vi "ccd_livescan.vi"(8 "Or, read path automatically from:":path, 9 "Manual save directory":string, 10 "Manual save path":path, 11 "Manual (up) or automatic (down)":bool) -> ()   [LabVIEW 2009]
uses:
  <vilib>/vision/NI_Vision_Development_Module.lvlib
panel:
  in  "STOP":bool
  out "Log":string
  out "RFPI":dbl
  out "YFPI":dbl
  out "GFPI":dbl
  out "CI":dbl
  out "RI":dbl
  out "GI":dbl
  out "BF":dbl
  out "Loop counter (not important)":i32
  out "Live saturation image":T1(plugin-control)
  out "Live image":T1(plugin-control)
  out "Histogram graph":T2(graph)
  out "Snapshots":string
  in  "Custom snapshot":bool
  in  "BF snapshot":bool
  in  "RFP snapshot":bool
  in  "YFP snapshot":bool
  in  "GFP snapshot":bool
  in  "Red snapshot":bool
  in  "Green snapshot":bool
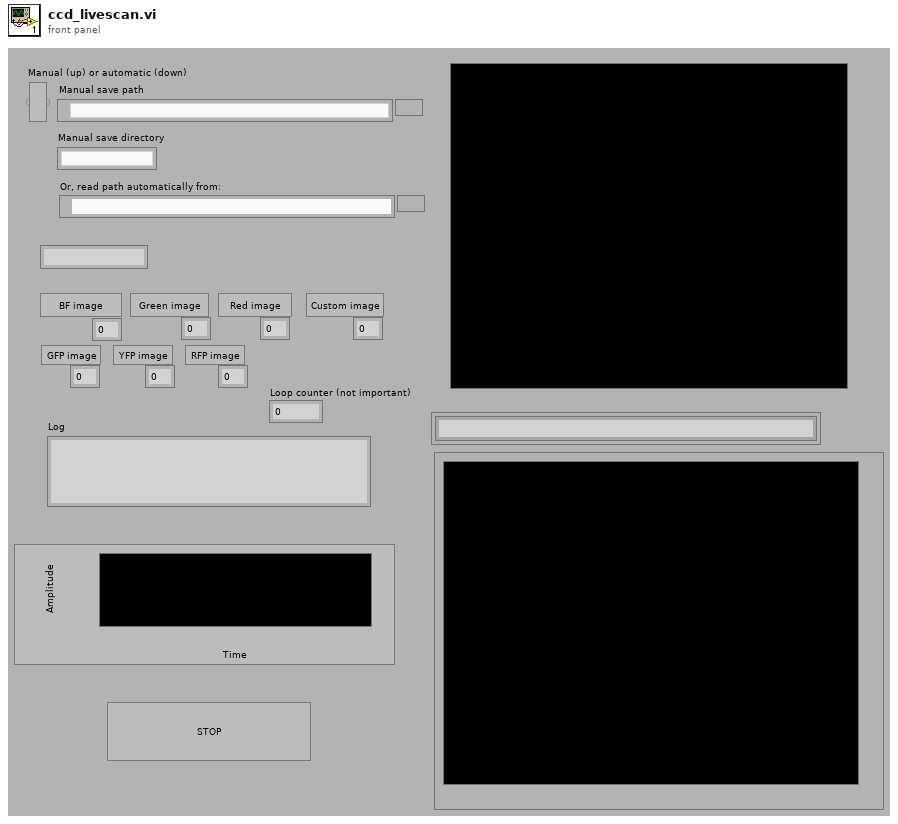
[diagram p1: front panel]
types:
  T1 = typedef "IMAQ Image.ctl" = refnum<image>
  T2 = cluster{"Starting Value":sgl, "Incremental Value":sgl, "Histogram":u32[]}
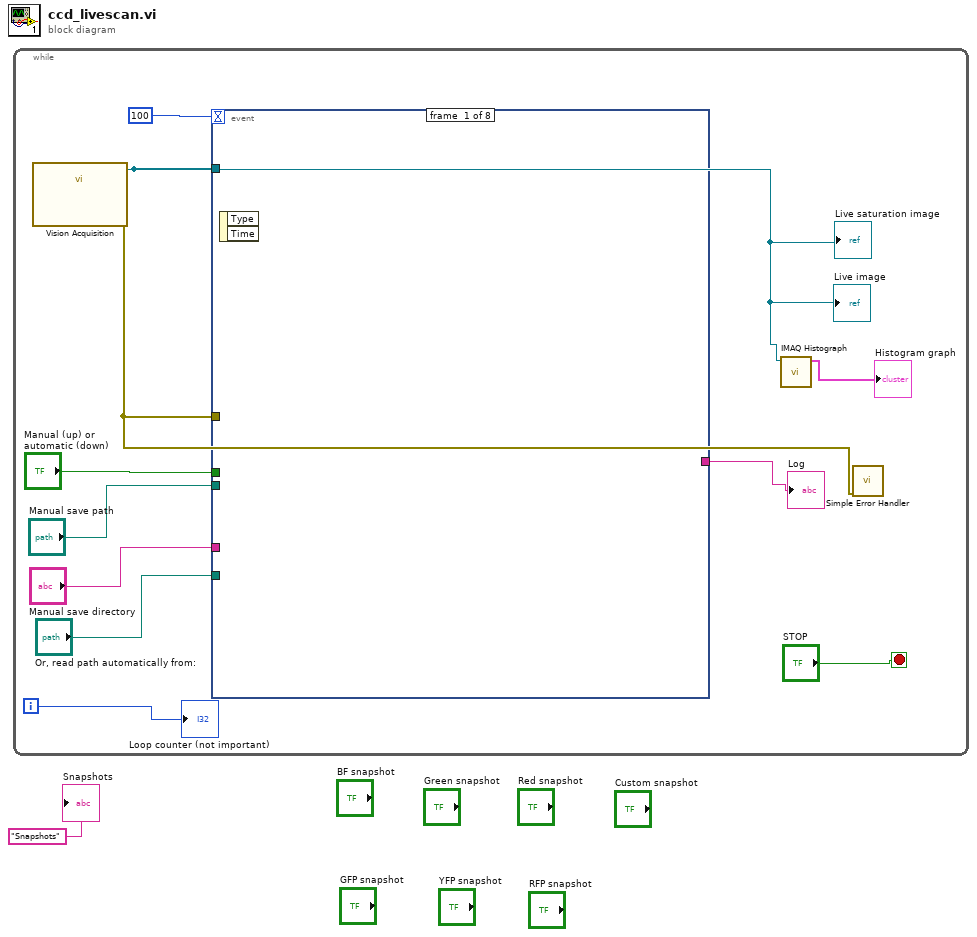
[diagram p0: block diagram]
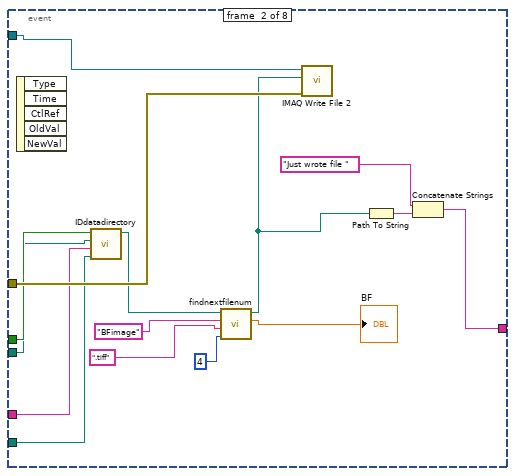
[diagram p2: hidden frame]
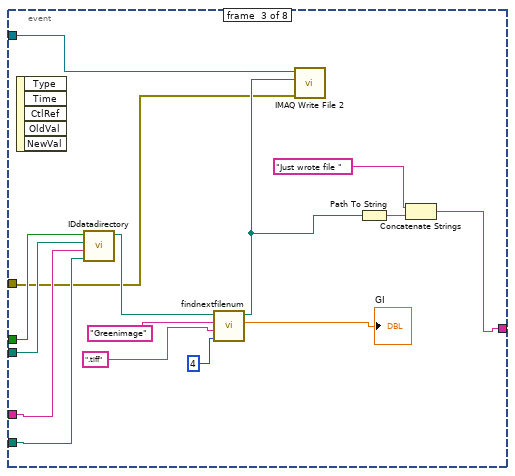
[diagram p3: hidden frame]
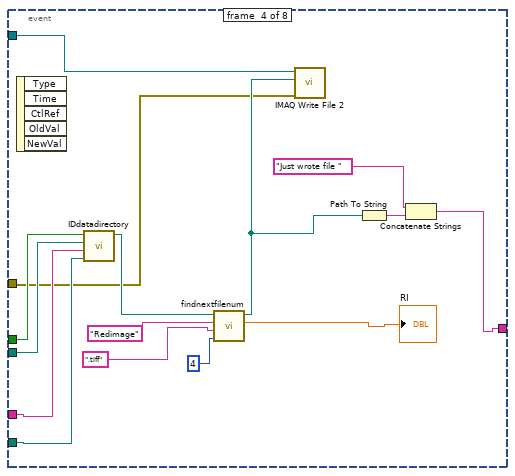
[diagram p4: hidden frame]
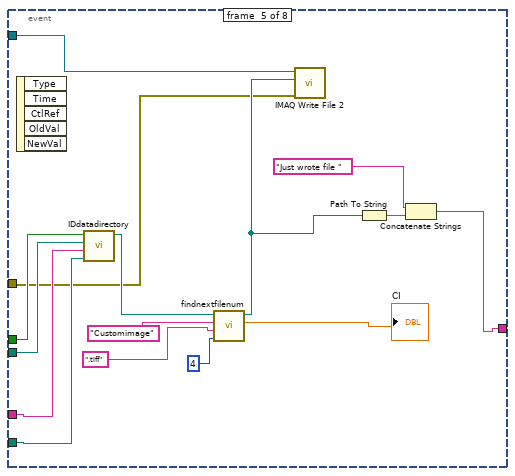
[diagram p5: hidden frame]
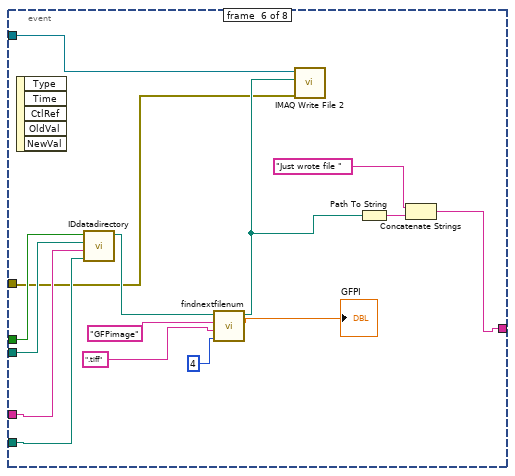
[diagram p6: hidden frame]
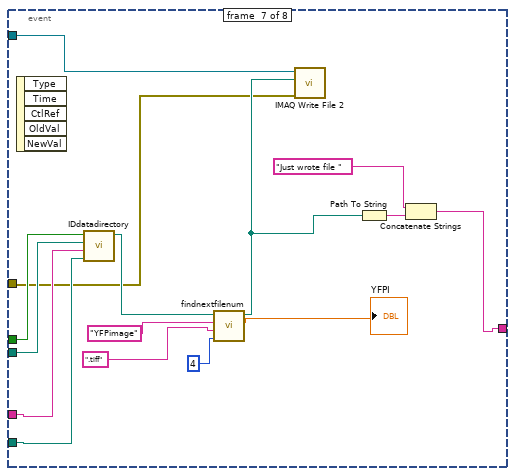
[diagram p7: hidden frame]
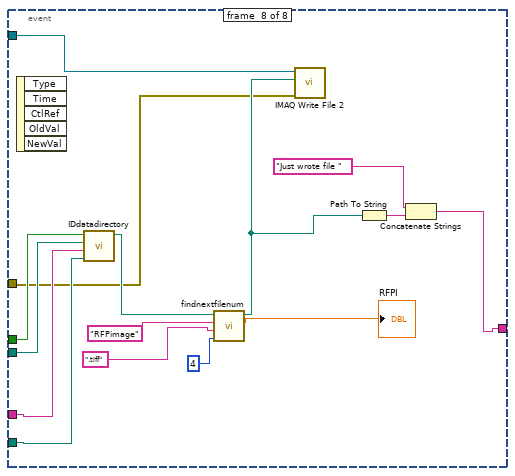
[diagram p8: hidden frame]
diagram:
  n1 = while {
    i -> [w12]
    stop <- "STOP" stop-if-true
    n2 = call "Vision Acquisition"() -> ("Image Out"=w8:T1, "error out"=w7:errorcluster)  [unwired: 25 in, 1 out]
    "Live saturation image" <- w8
    "Live image" <- w8
    n3 = event shown="[5] \"GFP snapshot\": Value Change" {
      selector: _ -> [_ _ _ _ _ _ _ _]
      dyn-events: _ -> [_ _ _ _ _ _ _ _]
      timeout: 100 -> [_ _ _ _ _ _ _ _]
      tunnel: "Manual save path" -> [_ w19 w33 w48 w63 w78 w93 w108]
      tunnel: w8 -> [_ w27 w30 w45 w60 w75 w90 w105]
      tunnel: w7 -> [_ w26 w31 w46 w61 w76 w91 w106]
      tunnel: "Manual save directory" -> [_ w18 w34 w49 w64 w79 w94 w109]
      tunnel: "Manual (up) or automatic (down)" -> [_ w20 w32 w47 w62 w77 w92 w107]
      tunnel: "Or, read path automatically from:" -> [_ w17 w35 w50 w65 w80 w95 w110]
      tunnel: [_ w14 w28 w44 w59 w74 w89 w104] -> w3
      event #0 {
        n4 = event-data() -> ()  [unwired: 1 in, 2 out]
      }
      event #1 {
        n5 = event-data() -> ()  [unwired: 1 in, 5 out]
        n6 = call "IDdatadirectory.vi"("Read path automatically from:"=w17, "Directory"=w18, "Save path"=w19, "Manual or automatic"=w20) -> ("Outputpath"=w15:path)  [unwired: 7 in]
        n7 = call "findnextfilenum.vi"("digits"=4, "extension"=".tiff", "filename"="BFimage", "Path"=w15) -> ("Output"=→"BF":dbl, "fulloutputpath"=w13:path)  [unwired: 4 in]
        n8 = call-poly "IMAQ Write File 2"("error in (no error)"=w26, "File Path"=w13, "Image"=w27) -> ()  [unwired: 7 in, 2 out]
        n9 = Path To String(path=w13) -> (string=w16:string)
        n10 = Concatenate Strings("Just wrote file ", w16) -> (w14:string)
      }
      event #2 {
        n11 = event-data() -> ()  [unwired: 1 in, 5 out]
        n12 = call "IDdatadirectory.vi"("Read path automatically from:"=w35, "Directory"=w34, "Save path"=w33, "Manual or automatic"=w32) -> ("Outputpath"=w37:path)  [unwired: 7 in]
        n13 = call "findnextfilenum.vi"("digits"=4, "extension"=".tiff", "filename"="Greenimage", "Path"=w37) -> ("Output"=→"GI":dbl, "fulloutputpath"=w36:path)  [unwired: 4 in]
        n14 = call-poly "IMAQ Write File 2"("error in (no error)"=w31, "File Path"=w36, "Image"=w30) -> ()  [unwired: 7 in, 2 out]
        n15 = Path To String(path=w36) -> (string=w38:string)
        n16 = Concatenate Strings("Just wrote file ", w38) -> (w28:string)
      }
      event #3 {
        n17 = event-data() -> ()  [unwired: 1 in, 5 out]
        n18 = call "IDdatadirectory.vi"("Read path automatically from:"=w50, "Directory"=w49, "Save path"=w48, "Manual or automatic"=w47) -> ("Outputpath"=w52:path)  [unwired: 7 in]
        n19 = call "findnextfilenum.vi"("digits"=4, "extension"=".tiff", "filename"="Redimage", "Path"=w52) -> ("Output"=→"RI":dbl, "fulloutputpath"=w51:path)  [unwired: 4 in]
        n20 = call-poly "IMAQ Write File 2"("error in (no error)"=w46, "File Path"=w51, "Image"=w45) -> ()  [unwired: 7 in, 2 out]
        n21 = Path To String(path=w51) -> (string=w53:string)
        n22 = Concatenate Strings("Just wrote file ", w53) -> (w44:string)
      }
      event #4 {
        n23 = event-data() -> ()  [unwired: 1 in, 5 out]
        n24 = call "IDdatadirectory.vi"("Read path automatically from:"=w65, "Directory"=w64, "Save path"=w63, "Manual or automatic"=w62) -> ("Outputpath"=w67:path)  [unwired: 7 in]
        n25 = call "findnextfilenum.vi"("digits"=4, "extension"=".tiff", "filename"="Customimage", "Path"=w67) -> ("Output"=→"CI":dbl, "fulloutputpath"=w66:path)  [unwired: 4 in]
        n26 = call-poly "IMAQ Write File 2"("error in (no error)"=w61, "File Path"=w66, "Image"=w60) -> ()  [unwired: 7 in, 2 out]
        n27 = Path To String(path=w66) -> (string=w68:string)
        n28 = Concatenate Strings("Just wrote file ", w68) -> (w59:string)
      }
      event #5 {
        n29 = event-data() -> ()  [unwired: 1 in, 5 out]
        n30 = call "IDdatadirectory.vi"("Read path automatically from:"=w80, "Directory"=w79, "Save path"=w78, "Manual or automatic"=w77) -> ("Outputpath"=w82:path)  [unwired: 7 in]
        n31 = call "findnextfilenum.vi"("digits"=4, "extension"=".tiff", "filename"="GFPimage", "Path"=w82) -> ("Output"=→"GFPI":dbl, "fulloutputpath"=w81:path)  [unwired: 4 in]
        n32 = call-poly "IMAQ Write File 2"("error in (no error)"=w76, "File Path"=w81, "Image"=w75) -> ()  [unwired: 7 in, 2 out]
        n33 = Path To String(path=w81) -> (string=w83:string)
        n34 = Concatenate Strings("Just wrote file ", w83) -> (w74:string)
      }
      event #6 {
        n35 = event-data() -> ()  [unwired: 1 in, 5 out]
        n36 = call "IDdatadirectory.vi"("Read path automatically from:"=w95, "Directory"=w94, "Save path"=w93, "Manual or automatic"=w92) -> ("Outputpath"=w97:path)  [unwired: 7 in]
        n37 = call "findnextfilenum.vi"("digits"=4, "extension"=".tiff", "filename"="YFPimage", "Path"=w97) -> ("Output"=→"YFPI":dbl, "fulloutputpath"=w96:path)  [unwired: 4 in]
        n38 = call-poly "IMAQ Write File 2"("error in (no error)"=w91, "File Path"=w96, "Image"=w90) -> ()  [unwired: 7 in, 2 out]
        n39 = Path To String(path=w96) -> (string=w98:string)
        n40 = Concatenate Strings("Just wrote file ", w98) -> (w89:string)
      }
      event #7 {
        n41 = event-data() -> ()  [unwired: 1 in, 5 out]
        n42 = call "IDdatadirectory.vi"("Read path automatically from:"=w110, "Directory"=w109, "Save path"=w108, "Manual or automatic"=w107) -> ("Outputpath"=w112:path)  [unwired: 7 in]
        n43 = call "findnextfilenum.vi"("digits"=4, "extension"=".tiff", "filename"="RFPimage", "Path"=w112) -> ("Output"=→"RFPI":dbl, "fulloutputpath"=w111:path)  [unwired: 4 in]
        n44 = call-poly "IMAQ Write File 2"("error in (no error)"=w106, "File Path"=w111, "Image"=w105) -> ()  [unwired: 7 in, 2 out]
        n45 = Path To String(path=w111) -> (string=w113:string)
        n46 = Concatenate Strings("Just wrote file ", w113) -> (w104:string)
      }
    }
    "Log" <- w3
    n47 = call "IMAQ Histograph"("Image"=w8) -> ("Histogram Graph"=→"Histogram graph":T2)  [unwired: 7 in, 3 out]
    n48 = call <vilib>:"Simple Error Handler.vi"("error in (no error)"=w7) -> ()  [unwired: 4 in, 5 out]
    "Loop counter (not important)" <- w12
  }
  "Snapshots" <- "Snapshots"
